vi "CRYProbe Window Update.vi"(8 "NamesforRename":string[](array[string]), 9 "ProbeType":string, 10 "sAction":string, 11 "Names":string[](array[string])) -> ()   [LabVIEW 2013]
uses:
  Global/CRYCurve Library Global.vi
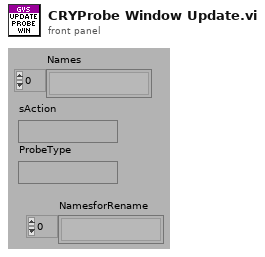
[diagram p1: front panel]
types:
  T1 = cluster{"Type Name":string, "Data Name":string, "Probe VIRef Number":i32, "Probe VIRef":refnum<vi>}[]
  T2 = cluster{"Type Name":string, "Data Name":string, "Probe VIRef Number":i32, "Probe VIRef":refnum<vi>}
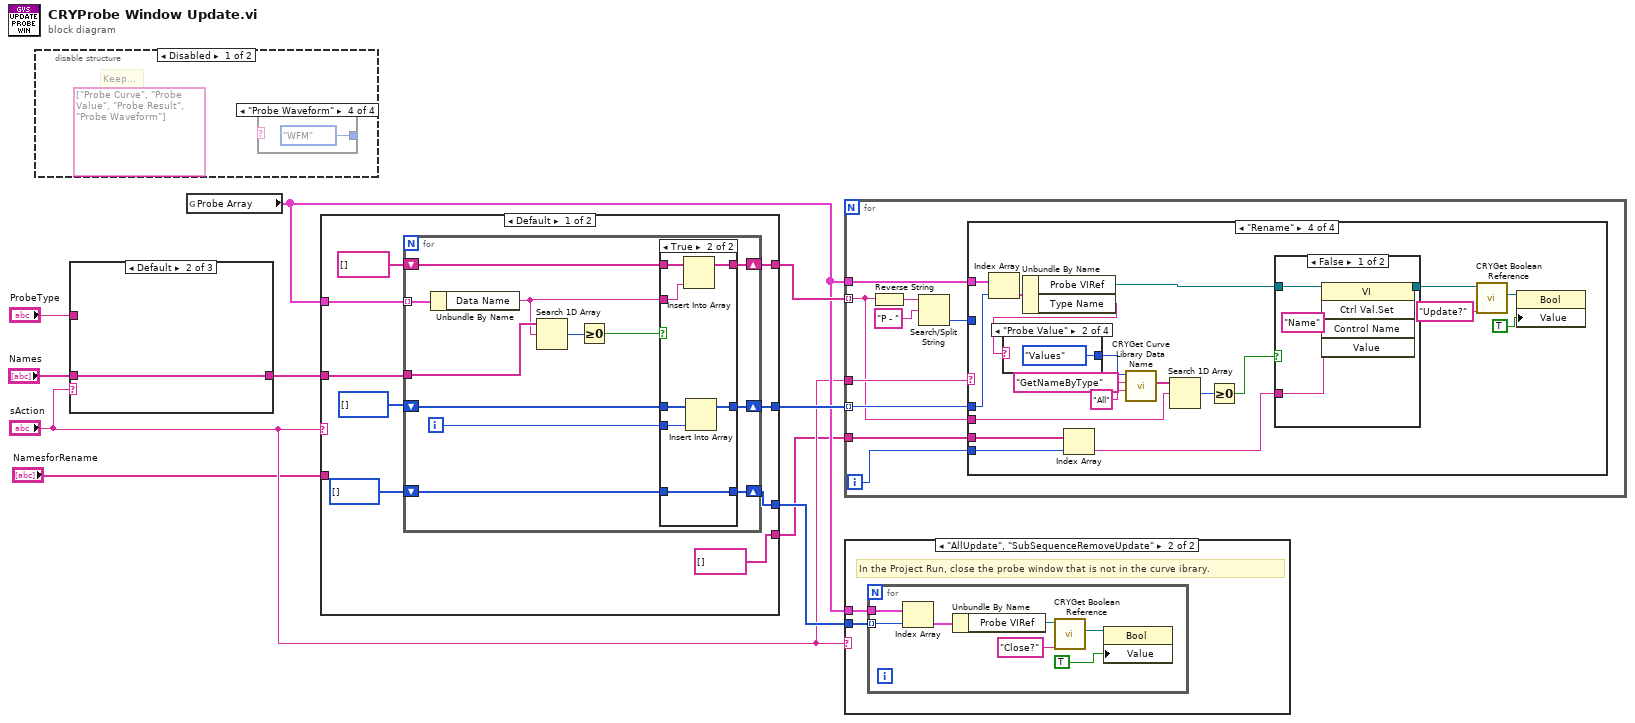
[diagram p0: block diagram]
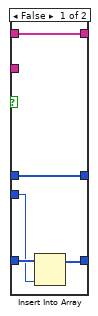
[diagram p2: hidden frame]
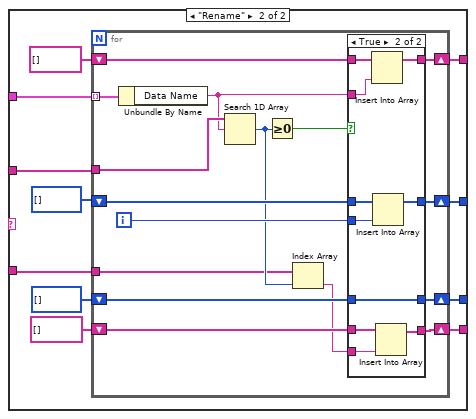
[diagram p3: hidden frame]
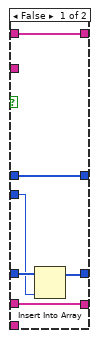
[diagram p4: hidden frame]
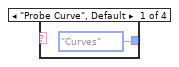
[diagram p5: hidden frame]
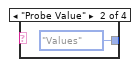
[diagram p6: hidden frame]
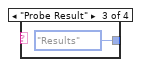
[diagram p7: hidden frame]
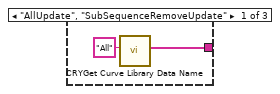
[diagram p10: hidden frame]
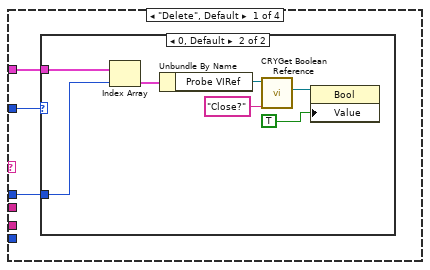
[diagram p12: hidden frame]
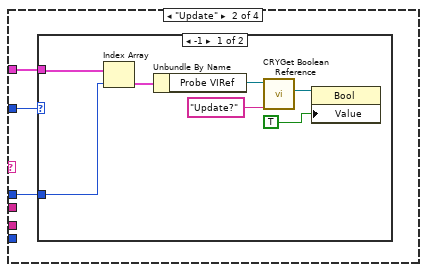
[diagram p14: hidden frame]
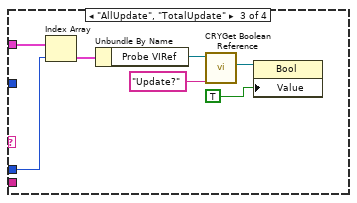
[diagram p16: hidden frame]
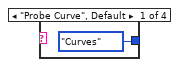
[diagram p17: hidden frame]
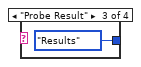
[diagram p18: hidden frame]
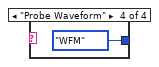
[diagram p19: hidden frame]
diagram:
  n1 = disable-structure shown="Disabled" {
    frame Disabled {
      (unwired) string[] ["Probe Curve", "Probe Value", "Probe Result", "Probe Waveform"]
      # "Keep..."
      n2 = case shown="\"Probe Waveform\"" {
        selector: _ -> [_ _ _ _]
        tunnel: [enum16{"Curves", "Values", "Results", "WFM"}."Curves" ("Type") enum16{"Curves", "Values", "Results", "WFM"}."Values" ("Type") enum16{"Curves", "Values", "Results", "WFM"}."Results" ("Type") enum16{"Curves", "Values", "Results", "WFM"}."WFM" ("Type")] -> _
        frame "Probe Curve", Default {
        }
        frame "Probe Value" {
        }
        frame "Probe Result" {
        }
        frame "Probe Waveform" {
        }
      }
    }
    frame Enabled {
    }
  }
  n3 = case shown="Default" "sAction" {
    tunnel: [w15 w17 w18] -> w8
    tunnel: "ProbeType" -> [_ _ _]
    tunnel: "Names" -> [_ w17 w18]
    frame "AllUpdate", "SubSequenceRemoveUpdate" {
      n4 = call "CRYGet Curve Library Data Name.vi"("sAction"="All") -> ("sNames"=w15:string[])  [unwired: 5 in, 5 out]
    }
    frame Default {
    }
    frame "Rename" {
    }
  }
  n5 = global read "CRYCurve Library Global.vi" "Probe Array"() -> (w6:T1)
  n6 = case shown="Default" "sAction" {
    tunnel: [w26 w61] -> w10
    tunnel: [w24 w59] -> w9
    tunnel: w8 -> [w23 w58]
    tunnel: w6 -> [w21 w56]
    tunnel: [w20 w55] -> w5
    tunnel: "NamesforRename" -> [_ w53]
    tunnel: [string[] [] w52] -> w1
    frame Default {
      n7 = for {
        tunnel: w21 -> [w39] mode=indexing
        shift-right: [w36] -> w26
        shift-left: i32[] [] ("Protected Array") -> [w38]
        tunnel: w23 -> [w35]
        shift-right: [w32] -> w24
        shift-left: string[] [] -> [w33]
        shift-right: [w29] -> w20
        shift-left: i32[] [] ("Protected Array") -> [w30]
        i -> [w37]
        n8 = Unbundle By Name(w39) -> ("Data Name"=w31:string)
        n9 = Search 1D Array(1D array=w35, element=w31) -> (index of element=w28:i32)  [unwired: 1 out]
        n10 = Greater Or Equal To 0?(x=w28) -> (x >= 0?=w34:bool)
        n11 = case shown="True" w34 {
          tunnel: w38 -> [w44 w51]
          tunnel: w37 -> [w40 w50]
          tunnel: [w44 w49] -> w36
          tunnel: [w43 w47] -> w32
          tunnel: w33 -> [w43 w48]
          tunnel: w31 -> [_ w46]
          tunnel: w30 -> [w42 w45]
          tunnel: [w41 w45] -> w29
          frame False {
            n12 = Insert Into Array(array=w42, new element=w40) -> (w41:i32[])  [unwired: 1 in]
          }
          frame True {
            n13 = Insert Into Array(array=w48, new element=w46) -> (w47:string[])  [unwired: 1 in]
            n14 = Insert Into Array(array=w51, new element=w50) -> (w49:i32[])  [unwired: 1 in]
          }
        }
      }
    }
    frame "Rename" {
      n15 = for {
        tunnel: w56 -> [w78] mode=indexing
        shift-right: [w75] -> w61
        shift-left: i32[] [] ("Protected Array") -> [w77]
        tunnel: w58 -> [w74]
        shift-right: [w71] -> w59
        shift-left: string[] [] -> [w72]
        shift-right: [w68] -> w55
        shift-left: i32[] [] ("Protected Array") -> [w69]
        shift-right: [w67] -> w52
        shift-left: string[] [] -> [w66]
        tunnel: w53 -> [w64]
        i -> [w76]
        n16 = Unbundle By Name(w78) -> ("Data Name"=w70:string)
        n17 = Search 1D Array(1D array=w74, element=w70) -> (index of element=w65:i32)  [unwired: 1 out]
        n18 = Greater Or Equal To 0?(x=w65) -> (x >= 0?=w73:bool)
        n19 = Index Array(array=w64, index=w65) -> (element=w63:string)
        n20 = case shown="True" w73 {
          tunnel: w77 -> [w84 w94]
          tunnel: w76 -> [w80 w93]
          tunnel: [w84 w92] -> w75
          tunnel: [w83 w90] -> w71
          tunnel: w72 -> [w83 w91]
          tunnel: w70 -> [_ w89]
          tunnel: w69 -> [w82 w88]
          tunnel: [w81 w88] -> w68
          tunnel: [w79 w87] -> w67
          tunnel: w66 -> [w79 w86]
          tunnel: w63 -> [_ w85]
          frame False {
            n21 = Insert Into Array(array=w82, new element=w80) -> (w81:i32[])  [unwired: 1 in]
          }
          frame True {
            n22 = Insert Into Array(array=w91, new element=w89) -> (w90:string[])  [unwired: 1 in]
            n23 = Insert Into Array(array=w94, new element=w93) -> (w92:i32[])  [unwired: 1 in]
            n24 = Insert Into Array(array=w86, new element=w85) -> (w87:string[])  [unwired: 1 in]
          }
        }
      }
    }
  }
  n25 = for {
    tunnel: w6 -> [w100]
    tunnel: w10 -> [w99] mode=indexing
    tunnel: w9 -> [w96] mode=indexing
    tunnel: "sAction" -> [w98]
    tunnel: w1 -> [w97]
    i -> [w95]
    n26 = Reverse String(1:w96) -> (0:w102:string)
    n27 = Search/Split String(string=w102, search string/char (-)="P - ") -> (offset of match=w103:i32)  [unwired: 3 out]
    n28 = case shown="\"Rename\"" w98 {
      tunnel: w103 -> [w106 w116 _ _]
      tunnel: w100 -> [w105 w114 w125 w145]
      tunnel: w99 -> [w104 w115 w124 w144]
      tunnel: w97 -> [_ _ _ w133]
      tunnel: w96 -> [_ _ _ w134]
      tunnel: w95 -> [_ _ _ w132]
      frame "Delete", Default {
        n29 = case shown="0, Default" w106 {
          tunnel: w105 -> [_ w112]
          tunnel: w104 -> [_ w111]
          frame -1 {
          }
          frame 0, Default {
            n30 = Index Array(array=w112, index=w111) -> (element=w110:T2)
            n31 = Unbundle By Name(w110) -> ("Probe VIRef"=w113:refnum<vi>)
            n32 = call "CRYGet Boolean Reference.vi"("Label Name"="Close?", "VI Refnum"=w113) -> ("Boolean Ref"=w108:refnum<vi>)  [unwired: 9 out]
            n33 = property class="Bool"(reference=w108, "Value"=TRUE) -> ()  [unwired: 1 in, 2 out]
          }
        }
      }
      frame "Update" {
        n34 = case shown="-1" w116 {
          tunnel: w114 -> [w118 _]
          tunnel: w115 -> [w117 _]
          frame -1 {
            n35 = Index Array(array=w118, index=w117) -> (element=w122:T2)
            n36 = Unbundle By Name(w122) -> ("Probe VIRef"=w123:refnum<vi>)
            n37 = call "CRYGet Boolean Reference.vi"("Label Name"="Update?", "VI Refnum"=w123) -> ("Boolean Ref"=w120:refnum<vi>)  [unwired: 9 out]
            n38 = property class="Bool"(reference=w120, "Value"=TRUE) -> ()  [unwired: 1 in, 2 out]
          }
          frame 0, Default {
          }
        }
      }
      frame "AllUpdate", "TotalUpdate" {
        n39 = Index Array(array=w125, index=w124) -> (element=w127:T2)
        n40 = Unbundle By Name(w127) -> ("Probe VIRef"=w126:refnum<vi>)
        n41 = call "CRYGet Boolean Reference.vi"("Label Name"="Update?", "VI Refnum"=w126) -> ("Boolean Ref"=w129:refnum<vi>)  [unwired: 9 out]
        n42 = property class="Bool"(reference=w129, "Value"=TRUE) -> ()  [unwired: 1 in, 2 out]
      }
      frame "Rename" {
        n43 = Index Array(array=w145, index=w144) -> (element=w146:T2)
        n44 = Unbundle By Name(w146) -> ("Probe VIRef"=w143:refnum<vi>, "Type Name"=w141:string)
        n45 = case shown="\"Probe Value\"" w141 {
          tunnel: [enum16{"Curves", "Values", "Results", "WFM"}."Curves" ("Type") enum16{"Curves", "Values", "Results", "WFM"}."Values" ("Type") enum16{"Curves", "Values", "Results", "WFM"}."Results" ("Type") enum16{"Curves", "Values", "Results", "WFM"}."WFM" ("Type")] -> w140
          frame "Probe Curve", Default {
          }
          frame "Probe Value" {
          }
          frame "Probe Result" {
          }
          frame "Probe Waveform" {
          }
        }
        n46 = Index Array(array=w133, index=w132) -> (element=w131:string)
        n47 = call "CRYGet Curve Library Data Name.vi"("sOption"="All", "sAction"="GetNameByType", "Type"=w140) -> ("sNames"=w137:string[])  [unwired: 5 in, 3 out]
        n48 = Search 1D Array(1D array=w137, element=w134) -> (index of element=w136:i32)  [unwired: 1 in]
        n49 = Greater Or Equal To 0?(x=w136) -> (x >= 0?=w135:bool)
        n50 = case shown="False" w135 {
          tunnel: w143 -> [w157 w158]
          tunnel: [w156 w158] -> w142
          tunnel: w131 -> [w154 _]
          frame False {
            n51 = invoke class="VI" method="Ctrl Val.Set"(reference=w157, "Control Name"="Name", "Value"=w154) -> (reference out=w156:refnum<vi>)  [unwired: 2 in, 4 out]
          }
          frame True {
          }
        }
        n52 = call "CRYGet Boolean Reference.vi"("Label Name"="Update?", "VI Refnum"=w142) -> ("Boolean Ref"=w148:refnum<vi>)  [unwired: 9 out]
        n53 = property class="Bool"(reference=w148, "Value"=TRUE) -> ()  [unwired: 1 in, 2 out]
      }
    }
  }
  n54 = case shown="\"AllUpdate\", \"SubSequenceRemoveUpdate\"" "sAction" {
    tunnel: w6 -> [_ w160]
    tunnel: w5 -> [_ w159]
    frame Default {
    }
    frame "AllUpdate", "SubSequenceRemoveUpdate" {
      # "In the Project Run, close the probe window that is not in the curve ibrary."
      n55 = for {
        tunnel: w160 -> [w162]
        tunnel: w159 -> [w161] mode=indexing
        n56 = Index Array(array=w162, index=w161) -> (element=w164:T2)
        n57 = Unbundle By Name(w164) -> ("Probe VIRef"=w163:refnum<vi>)
        n58 = call "CRYGet Boolean Reference.vi"("Label Name"="Close?", "VI Refnum"=w163) -> ("Boolean Ref"=w166:refnum<vi>)  [unwired: 9 out]
        n59 = property class="Bool"(reference=w166, "Value"=TRUE) -> ()  [unwired: 1 in, 2 out]
      }
    }
  }
